vi "Write Time Format.vi"(8 "error in (no error)":errorcluster, 10 "Time Format":string, 11 "Generic Logger in":refnum<class "Generic Logger.lvclass">) -> (0 "error out":errorcluster, 3 "Generic Logger out":refnum<class "Generic Logger.lvclass">)   [LabVIEW 2020, in "Logging.lvlib" / "Generic Logger.lvclass"]
uses:
  Generic Logger.lvclass
  Generic Logger.lvclass/Generic Logger.ctl
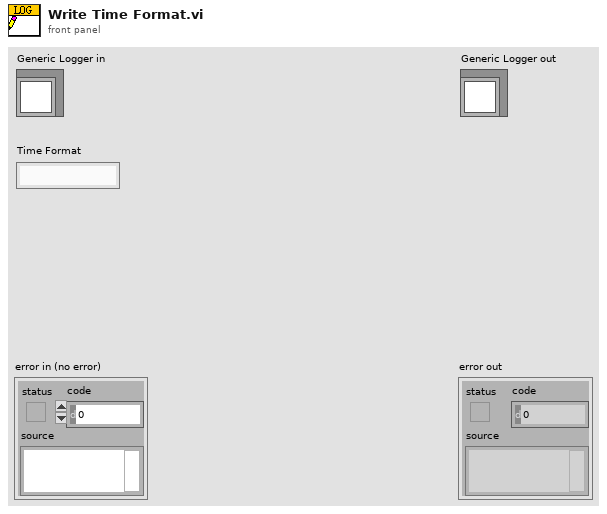
[diagram p1: front panel]
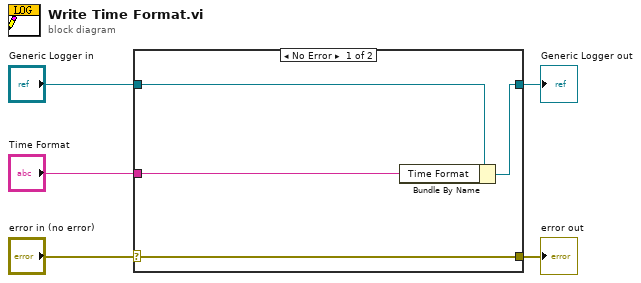
[diagram p0: block diagram]
diagram:
  n1 = case shown="No Error" "error in (no error)" {
    selector: "error in (no error)" -> [w9 w10]
    tunnel: [w9 w10] -> w4
    tunnel: [w7 w11] -> w2
    tunnel: "Generic Logger in" -> [w8 w11]
    tunnel: "Time Format" -> [w6 _]
    frame No Error {
      n2 = Bundle By Name(cluster=w8, "Time Format"=w6) -> (w7:refnum<class "Generic Logger.lvclass">)
    }
    frame Error {
    }
  }
  "error out" <- w4
  "Generic Logger out" <- w2
